vi "Graph_RMS_v00.vi"(6 "Inverse":bool, 8 "Min":T1, 9 "Max":T2, 10 "RMS Thresh":T3={"Pump A"=2, "Pump B"=0, "EPR"=40, "Graph"=0, "HD A"=40, "HD B"=0}, 11 "Cavity Errors":T4={"Pump A"=0, "Pump B"=1800, "EPR"=0, "Graph"=0, "HD A"=0, "HD B"=0}) -> (0 "UnlLocked?(T=yes)":cluster{bool, bool, bool, bool, bool, bool}, 1 "Unlocked?(T=Don`t measure)":bool)   [LabVIEW 2011]
doc: "Determines if a phase locked signal has crossed a user-defined threshold. Useful for comparing fluctuations that are normalised to RMS values."
uses:
  Strict Type Defs/Graph Errors.ctl
  Strict Type Defs/Lock Thresh Graph.ctl
  Strict Type Defs/Graph Max.ctl
  Strict Type Defs/Graph Min.ctl
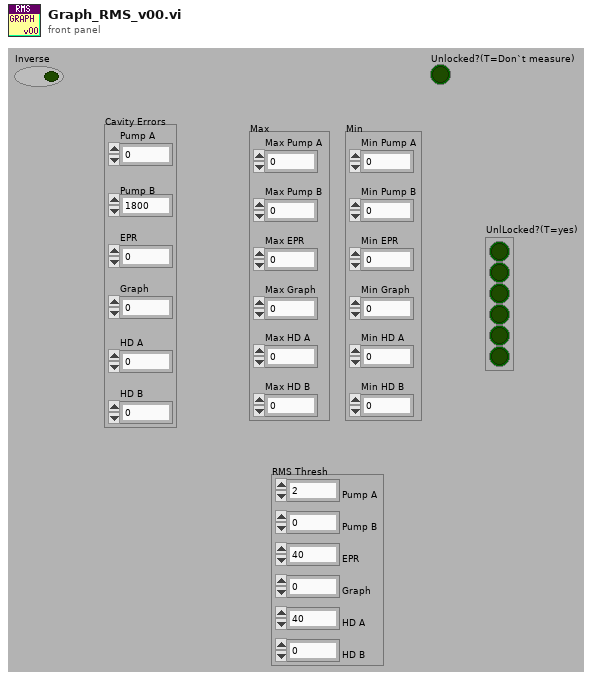
[diagram p1: front panel]
types:
  T1 = typedef "Graph Min.ctl" = cluster{"Min Pump A":i16, "Min Pump B":i16, "Min EPR":i16, "Min Graph":i16, "Min HD A":i16, "Min HD B":i16}
  T2 = typedef "Graph Max.ctl" = cluster{"Max Pump A":i16, "Max Pump B":i16, "Max EPR":i16, "Max Graph":i16, "Max HD A":i16, "Max HD B":i16}
  T3 = typedef "Lock Thresh Graph.ctl" = cluster{"Pump A":i16, "Pump B":i16, "EPR":i16, "Graph":i16, "HD A":i16, "HD B":i16}
  T4 = typedef "Graph Errors.ctl" = cluster{"Pump A":i16, "Pump B":i16, "EPR":i16, "Graph":i16, "HD A":i16, "HD B":i16}
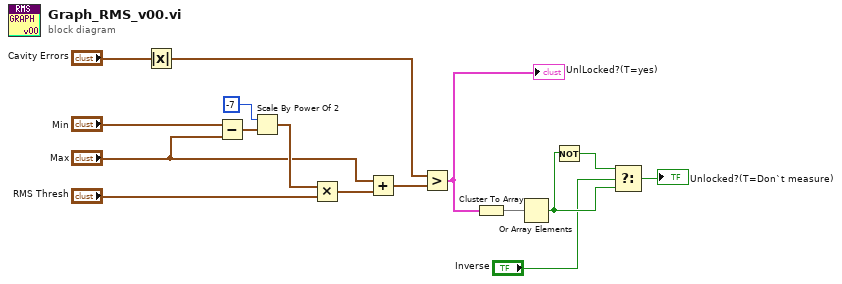
[diagram p0: block diagram]
diagram:
  n1 = Absolute Value(x="Cavity Errors") -> (abs(x)=w11:T4)
  n2 = Subtract(x="Min", y="Max") -> (x-y=w15:T1)
  n3 = Scale By Power Of 2(n=-7, x=w15) -> (x*2^n=w13:T1)
  n4 = Multiply(x=w13, y="RMS Thresh") -> (x*y=w14:T1)
  n5 = Add(x="Max", y=w14) -> (x+y=w12:T2)
  n6 = Greater?(x=w11, y=w12) -> (0:w6:cluster{bool, bool, bool, bool, bool, bool})
  "UnlLocked?(T=yes)" <- w6
  n7 = Cluster To Array(cluster=w6) -> (array=w5:bool[])
  n8 = Or Array Elements(Boolean array=w5) -> (logical OR=w3:bool)
  n9 = Not(x=w3) -> (.not. x?=w2:bool)
  n10 = Select(t=w2, s="Inverse", f=w3) -> (s? t:f=→"Unlocked?(T=Don`t measure)":bool)
